vi "connection type.vi"() -> (3 "connection type":T1=enum."server")   [LabVIEW 2014, in "tcp server connection.lvclass"]
uses:
  tcp server connection.lvclass
  typedefs/connection type.ctl
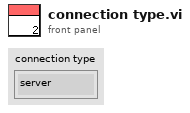
[diagram p1: front panel]
types:
  T1 = typedef "connection type.ctl" = enum16{"client", "server"}
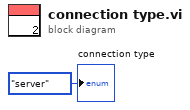
[diagram p0: block diagram]
diagram:
  "connection type" <- connection_type."server" ("connection type")
